vi "Word_Set_Scale.vi"(0 "Axes in":refnum<k7>, 5 "Type":i32(ring)=1 items=["xlCategory"=1, "xlSeriesAxis"=3, "xlValue"=2], 11 "error in":errorcluster, 12 "axis config":T1={"autoscale"=FALSE, "min"=0.0, "max"=0.0, "scale type"=-4132} {"scale type" items=["xlScaleLinear"=-4132, "xlScaleLogarithmic"=-4133]; "max" format="%.2f"; "min" format="%.2f"}) -> (4 "Axes out":refnum<k7>, 15 "error out":errorcluster)   [LabVIEW 2010, in "NI_ReportGenerationToolkit.lvlib"]
uses:
  <vilib>/addons/_office/NI_ReportGenerationToolkit.lvlib
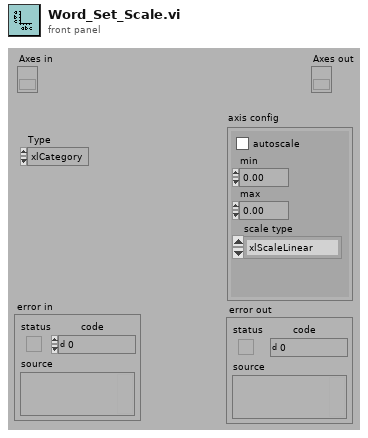
[diagram p1: front panel]
types:
  T1 = cluster{"autoscale":bool, "min":dbl, "max":dbl, "scale type":i32}
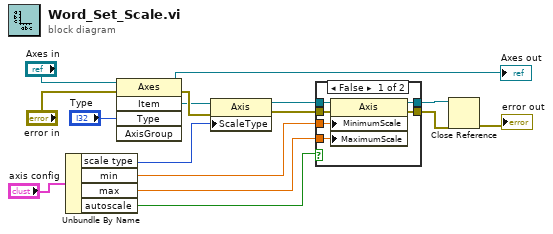
[diagram p0: block diagram]
diagram:
  n1 = Unbundle By Name("axis config") -> ("scale type"=w15:i32, "min"=w5:dbl, "max"=w4:dbl, "autoscale"=w3:bool)
  n2 = invoke class="Axes" method="Item"(reference="Axes in", error in="error in", "Type"="Type") -> (reference out=→"Axes out":refnum<k7>, error out=w13:errorcluster, "Item"=w11:refnum<k7>)  [unwired: 2 in, 2 out]
  n3 = property class="Axis"(reference=w11, error in=w13, "ScaleType"=w15) -> (reference out=w8:refnum<k7>, error out=w6:errorcluster)
  n4 = case shown="False" w3 {
    tunnel: w8 -> [w22 w24]
    tunnel: [w21 w24] -> w7
    tunnel: w6 -> [w20 w23]
    tunnel: [w19 w23] -> w1
    tunnel: w5 -> [w18 _]
    tunnel: w4 -> [w17 _]
    frame False {
      n5 = property class="Axis"(reference=w22, error in=w20, "MinimumScale"=w18, "MaximumScale"=w17) -> (reference out=w21:refnum<k7>, error out=w19:errorcluster)
    }
    frame True {
    }
  }
  n6 = Close Reference(reference=w7, error in (no error)=w1) -> (error out=→"error out":errorcluster)
